vi "pos_motor2encoder.vi"(8 "error in (no error)":errorcluster, 10 "pos in motor (pulses)":dbl, 11 "Motor in":refnum<class "Motor.lvclass">) -> (0 "error out":errorcluster, 2 "encoder unit":dbl, 3 "Motor out":refnum<class "Motor.lvclass">)   [LabVIEW 2016, in "Hardware.lvlib" / "Motor.lvlib" / "Motor.lvclass"]
uses:
  <userlib>/Common Components/Hardware/Motor/Motor/Motor.lvclass
  <userlib>/Common Components/Hardware/Motor/Motor/Motor.lvclass/Motor.ctl
  <userlib>/Common Components/Hardware/Motor/Motor/Accessor/Read encoder units ratio.vi
  <userlib>/Common Components/Hardware/Motor/Motor/Accessor/Read encoder type.vi
  <userlib>/Common Components/Hardware/Motor/Motor/Accessor/Read display units per motor rev.vi
  <userlib>/Common Components/Hardware/Motor/Motor/Accessor/Read motor pulses per revolution.vi
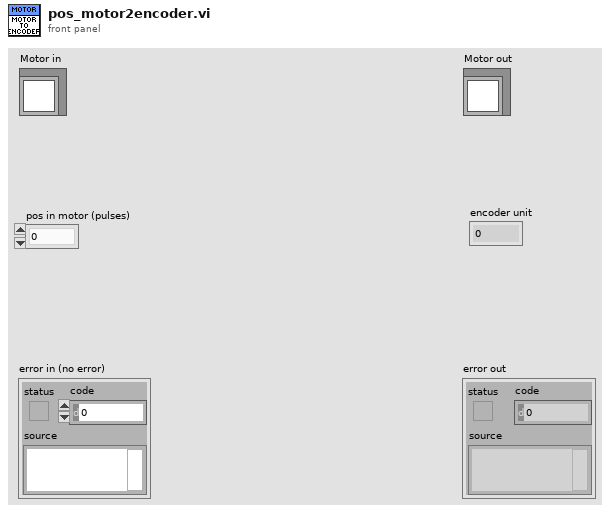
[diagram p1: front panel]
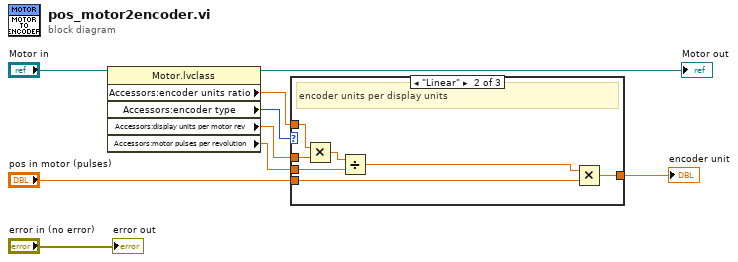
[diagram p0: block diagram]
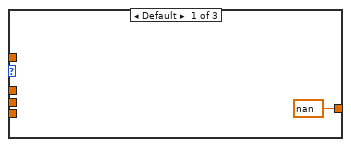
[diagram p2: hidden frame]
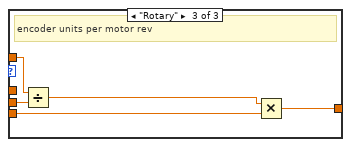
[diagram p3: hidden frame]
diagram:
  n1 = property class="Motor.lvclass"(reference="Motor in") -> (reference out=→"Motor out":refnum<class "Motor.lvclass">, "Accessors:encoder units ratio"=w5:dbl, "Accessors:encoder type"=w6:enum16{"Linear", "Rotary"}, "Accessors:display units per motor rev"=w4:dbl, "Accessors:motor pulses per revolution"=w3:dbl)  [unwired: 1 in, 1 out]
  n2 = case shown="\"Linear\"" w6 {
    tunnel: w5 -> [_ w17 w22]
    tunnel: w4 -> [_ w16 _]
    tunnel: w3 -> [_ w14 w21]
    tunnel: "pos in motor (pulses)" -> [_ w12 w20]
    tunnel: [nan ("Accessors:encoder units ratio") w11 w18] -> w1
    frame Default {
    }
    frame "Linear" {
      # "encoder units per display units"
      n3 = Multiply(x=w17, y=w16) -> (x*y=w15:dbl)
      n4 = Divide(x=w15, y=w14) -> (x/y=w13:dbl)
      n5 = Multiply(x=w13, y=w12) -> (x*y=w11:dbl)
    }
    frame "Rotary" {
      # "encoder units per motor rev"
      n6 = Divide(x=w22, y=w21) -> (x/y=w19:dbl)
      n7 = Multiply(x=w19, y=w20) -> (x*y=w18:dbl)
    }
  }
  "encoder unit" <- w1
  "error out" <- "error in (no error)"
